vi "Periodic Tasks.vi"(8 "error in":errorcluster) -> ()   [LabVIEW 2017]
doc: "This VI runs in parallel to other tasks. It can contain as many user-defined periodic loops as you need. These can carry out PID or other sorts of timed response."
uses:
  <vilib>/Rock Robotics/Network Tables/NT Read Number.vi
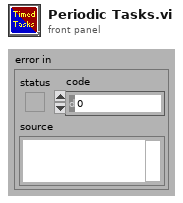
[diagram p1: front panel]
types:
  T1 = typedef "WPI_MotorControlDeviceRef.ctl" = cluster{"DeviceStatus":errorcluster, "Type":T2, "PWM":cluster{"PWM Channel":T3, "DeadBand":T4}, "CAN":cluster{"Device Number":u8, "SetOutput VI Ref":variant, "GetOutput VI Ref":variant, "Enable VI Ref":variant, "Disable VI Ref":variant, "Data":variant}, "Invert":bool, "DIO PWM":cluster{"PWM \"Enable\" Channel":T3, "DIOChannel":T5, "PWM Rate":dbl}}
  T2 = typedef "WPI_MotorControlType.ctl" = enum16{"PWM", "CAN", "DIO PWM"}
  T3 = typedef "FPGA_DIOPWMChannel.ctl" = enum8{"PWM 0", "PWM 1", "PWM 2", "PWM 3", "PWM 4", "PWM 5", "PWM 6", "PWM 7", "PWM 8", "PWM 9", "PWM MXP 0", "PWM MXP 1", "PWM MXP 2", "PWM MXP 3", "PWM MXP 4", "PWM MXP 5", "PWM MXP 6", "PWM MXP 7", "PWM MXP 8", "PWM MXP 9", "Invalid"}
  T4 = typedef "WPI_PWMDeadband.ctl" = cluster{"Name":string, "maxPositivePwm":i32, "minPositivePwm":i32, "centerPwm":i32, "maxNegativePwm":i32, "minNegativePwm":i32, "angularRange":u16}
  T5 = typedef "FPGA_DIOChannel.ctl" = enum8{"DIO 0", "DIO 1", "DIO 2", "DIO 3", "DIO 4", "DIO 5", "DIO 6", "DIO 7", "DIO 8", "DIO 9", "DIO MXP 0", "DIO MXP 1", "DIO MXP 2", "DIO MXP 3", "DIO MXP 4", "DIO MXP 5", "DIO MXP 6", "DIO MXP 7", "DIO MXP 8", "DIO MXP 9", "DIO MXP 10", "DIO MXP 11", "DIO MXP 12", "DIO MXP 13", "DIO MXP 14", "DIO MXP 15", "SPI Port CS1", "SPI Port CS2", "SPI Port CS3", "SPI Port MISO", "SPI Port MOSI", "Invalid"}
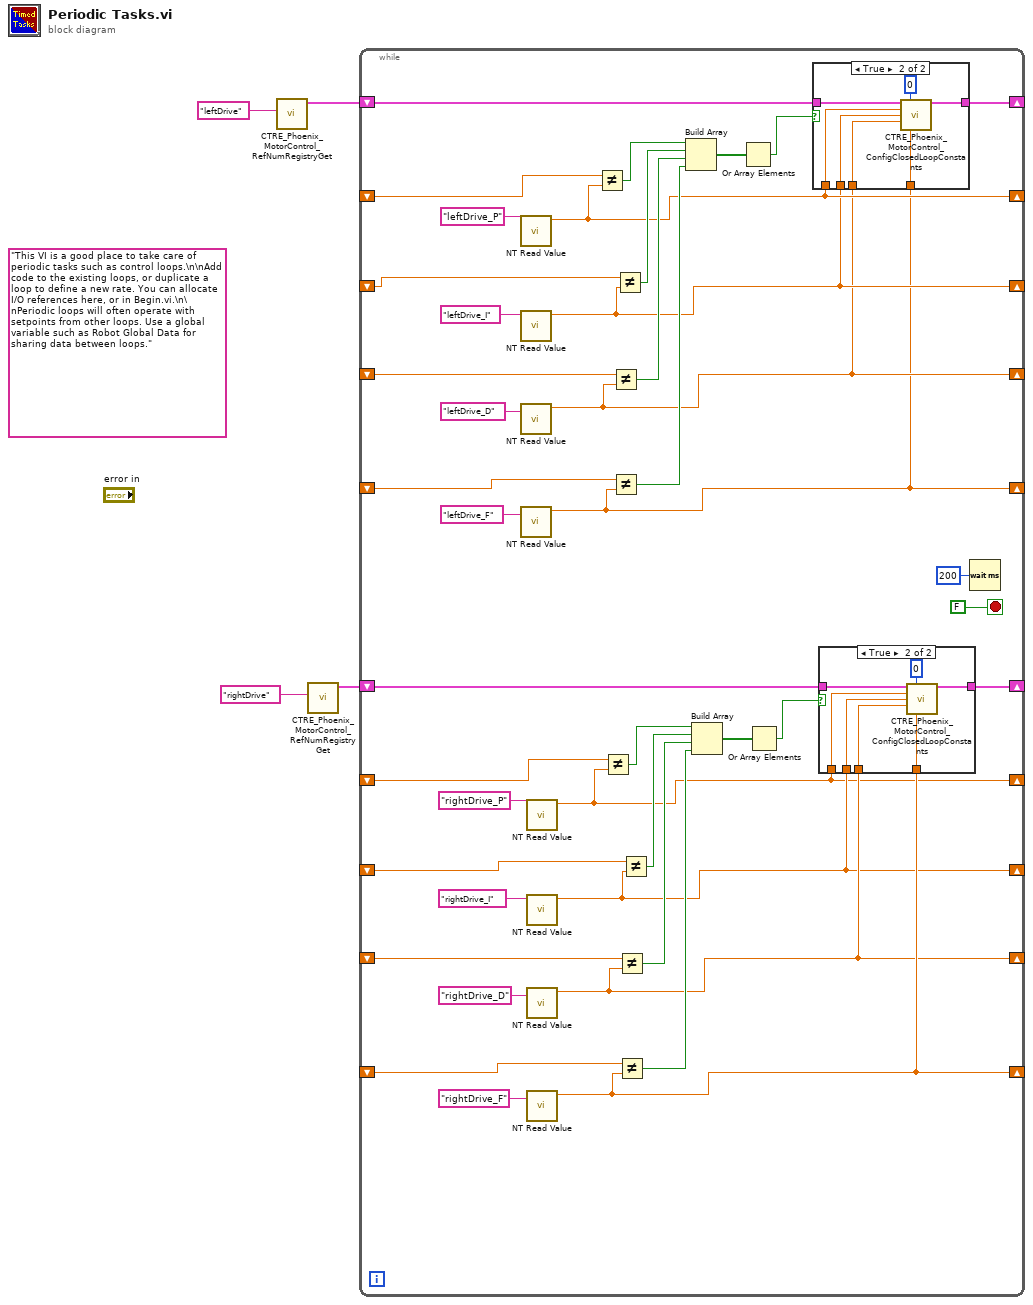
[diagram p0: block diagram]
diagram:
  (unwired) "This VI is a good place to take care of periodic tasks such as control loops.\n\nAdd code to the existing loops, or duplicate a loop to define a new rate. You can allocate I/O references here, or in Begin.vi.\n\nPeriodic loops will often operate with setpoints from other loops. Use a global variable such as Robot Global Data for sharing data between loops."
  n1 = call <vilib>:"CTRE_Phoenix_MotorControl_RefNumRegistryGet.vi"("refnum name"="leftDrive") -> ("PhoenixMotorControlDevRef"=w3:T1)  [unwired: 9 in, 1 out]
  n2 = call <vilib>:"CTRE_Phoenix_MotorControl_RefNumRegistryGet.vi"("refnum name"="rightDrive") -> ("PhoenixMotorControlDevRef"=w1:T1)  [unwired: 9 in, 1 out]
  n3 = while {
    shift-right: [w39] -> _
    shift-left: w3 -> [w40]
    shift-right: [w25] -> _
    shift-left: _ -> [w33]
    shift-right: [w26] -> _
    shift-left: _ -> [w32]
    shift-right: [w27] -> _
    shift-left: _ -> [w34]
    shift-right: [w28] -> _
    shift-left: _ -> [w35]
    shift-right: [w13] -> _
    shift-left: w1 -> [w14]
    shift-right: [w8] -> _
    shift-left: _ -> [w9]
    shift-right: [w7] -> _
    shift-left: _ -> [w10]
    shift-right: [w6] -> _
    shift-left: _ -> [w11]
    shift-right: [w5] -> _
    shift-left: _ -> [w12]
    stop <- FALSE stop-if-true
    n4 = call-poly <vilib>:"NT Read Value.vi"("Name"="leftDrive_P") -> ("Numeric"=w28:dbl)  [unwired: 9 in, 1 out]
    n5 = call-poly <vilib>:"NT Read Value.vi"("Name"="leftDrive_I") -> ("Numeric"=w27:dbl)  [unwired: 9 in, 1 out]
    n6 = call-poly <vilib>:"NT Read Value.vi"("Name"="leftDrive_D") -> ("Numeric"=w26:dbl)  [unwired: 9 in, 1 out]
    n7 = call-poly <vilib>:"NT Read Value.vi"("Name"="leftDrive_F") -> ("Numeric"=w25:dbl)  [unwired: 9 in, 1 out]
    n8 = call-poly <vilib>:"NT Read Value.vi"("Name"="rightDrive_P") -> ("Numeric"=w5:dbl)  [unwired: 9 in, 1 out]
    n9 = call-poly <vilib>:"NT Read Value.vi"("Name"="rightDrive_I") -> ("Numeric"=w6:dbl)  [unwired: 9 in, 1 out]
    n10 = call-poly <vilib>:"NT Read Value.vi"("Name"="rightDrive_D") -> ("Numeric"=w7:dbl)  [unwired: 9 in, 1 out]
    n11 = call-poly <vilib>:"NT Read Value.vi"("Name"="rightDrive_F") -> ("Numeric"=w8:dbl)  [unwired: 9 in, 1 out]
    n12 = Not Equal?(x=w35, y=w28) -> (x != y?=w36:bool)
    n13 = Not Equal?(x=w12, y=w5) -> (x != y?=w18:bool)
    n14 = Not Equal?(x=w32, y=w26) -> (x != y?=w30:bool)
    n15 = Not Equal?(x=w33, y=w25) -> (x != y?=w29:bool)
    n16 = Not Equal?(x=w34, y=w27) -> (x != y?=w31:bool)
    n17 = Not Equal?(x=w10, y=w7) -> (x != y?=w16:bool)
    n18 = Not Equal?(x=w9, y=w8) -> (x != y?=w15:bool)
    n19 = Not Equal?(x=w11, y=w6) -> (x != y?=w17:bool)
    n20 = Build Array(w36, w31, w30, w29) -> (w37:bool[])
    n21 = Build Array(w18, w17, w16, w15) -> (w19:bool[])
    n22 = Or Array Elements(Boolean array=w37) -> (logical OR=w38:bool)
    n23 = Or Array Elements(Boolean array=w19) -> (logical OR=w20:bool)
    n24 = case shown="True" w38 {
      tunnel: w40 -> [w55 w61]
      tunnel: [w55 w60] -> w39
      tunnel: w28 -> [_ w59]
      tunnel: w27 -> [_ w58]
      tunnel: w26 -> [_ w57]
      tunnel: w25 -> [_ w56]
      frame False {
      }
      frame True {
        n25 = call <vilib>:"CTRE_Phoenix_MotorControl_ConfigClosedLoopConstants.vi"("PhoenixMotorControlDevRef"=w61, "slotIdx"=0, "P"=w59, "I"=w58, "D"=w57, "F"=w56) -> ("PhoenixMotorControlDevRef"=w60:T1)  [unwired: 8 in, 1 out]
      }
    }
    n26 = case shown="True" w20 {
      tunnel: w14 -> [w47 w53]
      tunnel: [w47 w52] -> w13
      tunnel: w5 -> [_ w51]
      tunnel: w6 -> [_ w50]
      tunnel: w7 -> [_ w49]
      tunnel: w8 -> [_ w48]
      frame False {
      }
      frame True {
        n27 = call <vilib>:"CTRE_Phoenix_MotorControl_ConfigClosedLoopConstants.vi"("PhoenixMotorControlDevRef"=w53, "slotIdx"=0, "P"=w51, "I"=w50, "D"=w49, "F"=w48) -> ("PhoenixMotorControlDevRef"=w52:T1)  [unwired: 8 in, 1 out]
      }
    }
    n28 = Wait (ms)(milliseconds to wait=u32 200) -> ()  [unwired: 1 out]
  }
